vi "Stream Length.vi"(8 "error in (no error)":errorcluster, 11 "File Response in":refnum<class "File Response.lvclass">) -> (0 "error out":errorcluster, 2 "Length":i64, 3 "File Response out":refnum<class "File Response.lvclass">)   [LabVIEW 2020, in "HTTP Utils.lvlib" / "File Response.lvclass"]
uses:
  File Response.lvclass
  File Response.lvclass/File Response.ctl
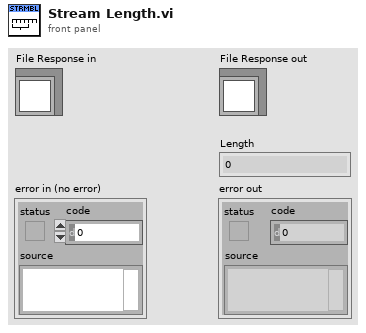
[diagram p1: front panel]
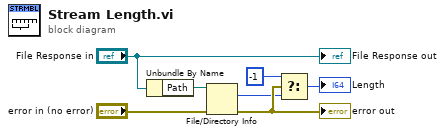
[diagram p0: block diagram]
diagram:
  n1 = Unbundle By Name("File Response in") -> ("Path"=w5:path)
  n2 = File/Directory Info(path=w5, error in="error in (no error)") -> (size=w3:i64, error out=w7:errorcluster)  [unwired: 5 out]
  "error out" <- w7
  n3 = Select(t=i64 -1, s=w7, f=w3) -> (s? t:f=→"Length":i64)
  "File Response out" <- "File Response in"
